vi "国标仪器获取加标回收数据.vi"(8 "error in (no error)":errorcluster, 11 "站号":u16(ring)=3 items=["总磷"=1, "总氮"=2, "氨氮"=3, "CODMn"=21, "CODCr"=22]) -> (0 "error out":errorcluster, 3 "测量数据区":T1)   [LabVIEW 2016, in "质控单元V1.lvlib"]
uses:
  <vilib>/Plasmionique/MB Master/MB_Master/MB_Master.lvclass
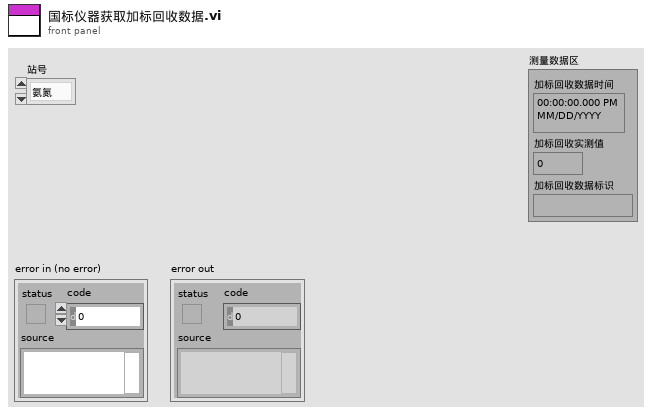
[diagram p1: front panel]
types:
  T1 = cluster{"加标回收数据时间":timestamp, "加标回收实测值":sgl, "加标回收数据标识":string}
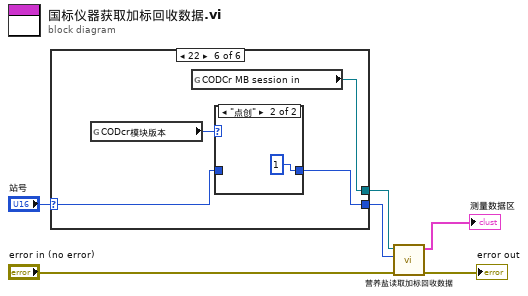
[diagram p0: block diagram]
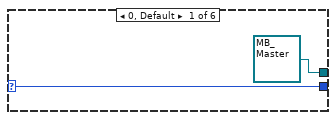
[diagram p2: hidden frame]
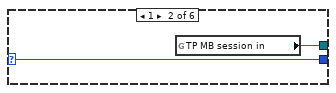
[diagram p3: hidden frame]
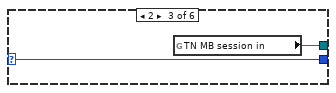
[diagram p4: hidden frame]
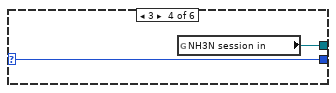
[diagram p5: hidden frame]
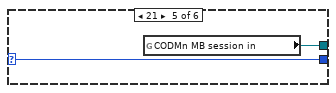
[diagram p6: hidden frame]
diagram:
  n1 = case shown="22" "站号" {
    selector: "站号" -> [w7 w9 w11 w13 w15 w18]
    tunnel: [refnum<class "MB_Master.lvclass"> refnum ("CODMn MB session in") w10 w12 w14 w16 w20] -> w6
    tunnel: [w7 w9 w11 w13 w15 w17] -> w1
    frame 0, Default {
    }
    frame 1 {
      n2 = global read "系统交互.vi" "TP MB session in"() -> (w10:refnum<class "MB_Master.lvclass">)
    }
    frame 2 {
      n3 = global read "系统交互.vi" "TN MB session in"() -> (w12:refnum<class "MB_Master.lvclass">)
    }
    frame 3 {
      n4 = global read "系统交互.vi" "NH3N session in"() -> (w14:refnum<class "MB_Master.lvclass">)
    }
    frame 21 {
      n5 = global read "系统交互.vi" "CODMn MB session in"() -> (w16:refnum<class "MB_Master.lvclass">)
    }
    frame 22 {
      n6 = global read "系统交互.vi" "CODcr模块版本"() -> (w19:enum16{"斯坦道V3", "点创"})
      n7 = global read "系统交互.vi" "CODCr MB session in"() -> (w20:refnum<class "MB_Master.lvclass">)
      n8 = case shown="\"点创\"" w19 {
        tunnel: w18 -> [w21 _]
        tunnel: [w21 u16 1 ("站号")] -> w17
        frame "斯坦道V3", Default {
        }
        frame "点创" {
        }
      }
    }
  }
  n9 = call "营养盐读取加标回收数据.vi"("error in (no error)"="error in (no error)", "站号"=w1, "MB session in"=w6) -> ("error out"=→"error out":errorcluster, "测量数据区"=→"测量数据区":T1)  [unwired: 7 in]
